vi "main.vi"() -> ()   [LabVIEW 2016]
uses:
  <vilib>/Analysis/baseanly.llb/Mean (DBL).vi
  <vilib>/Instr/_visa.llb/VISA Configure Serial Port (Instr).vi
  <vilib>/measure/mamon.llb/Waveform Peak Detection for 1 Chan.vi
  <vilib>/measure/NI_MAPro.lvlib
  <vilib>/Analysis/NI_AALBase.lvlib
panel:
  out "Heart Rate":string
  in  "Force Redraw":bool
  out "read buffer":string
  out "error out":errorcluster
  out "Value of last sample":i32
  out "Heart Rate Plot":i32(graph)
  out "Main loop interations":i32
  in  "stop":bool
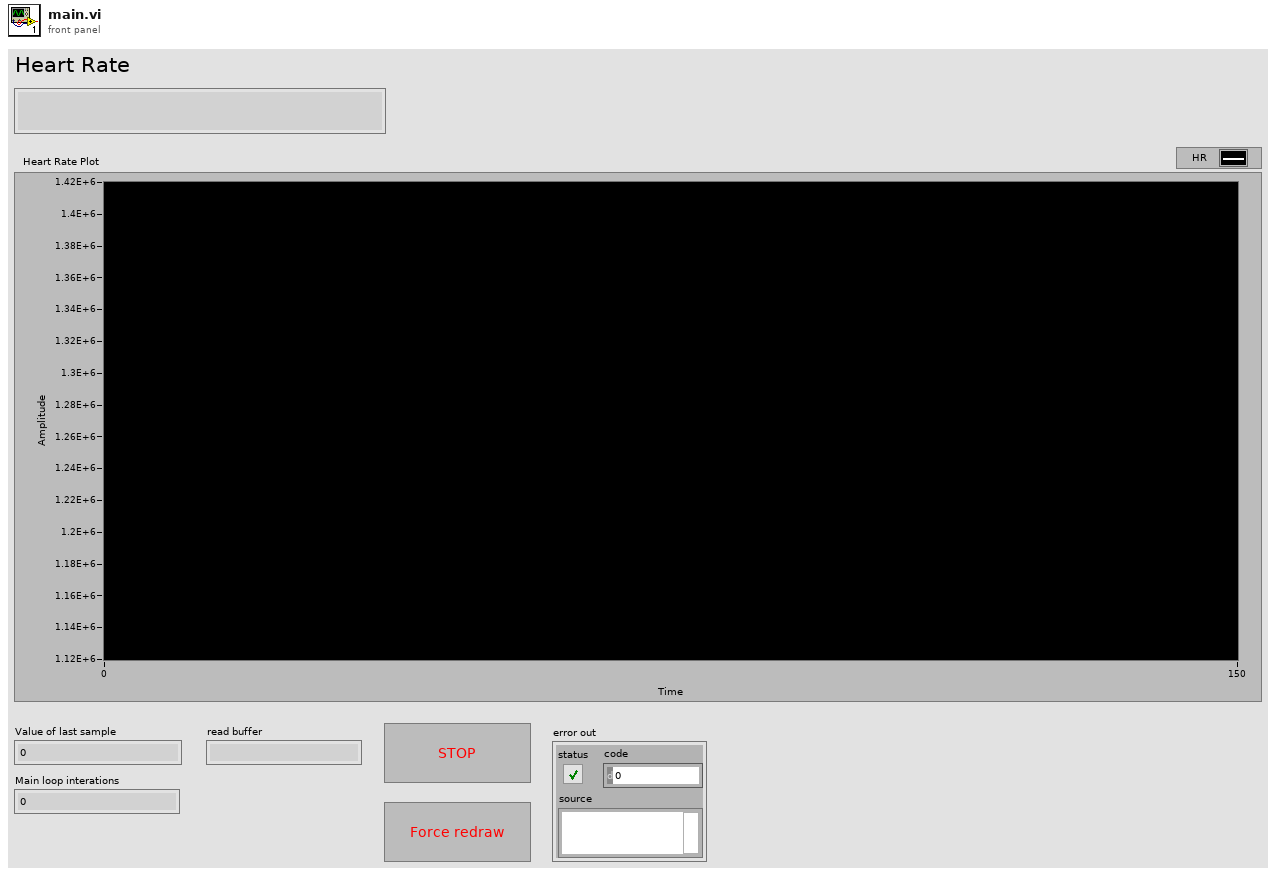
[diagram p1: front panel]
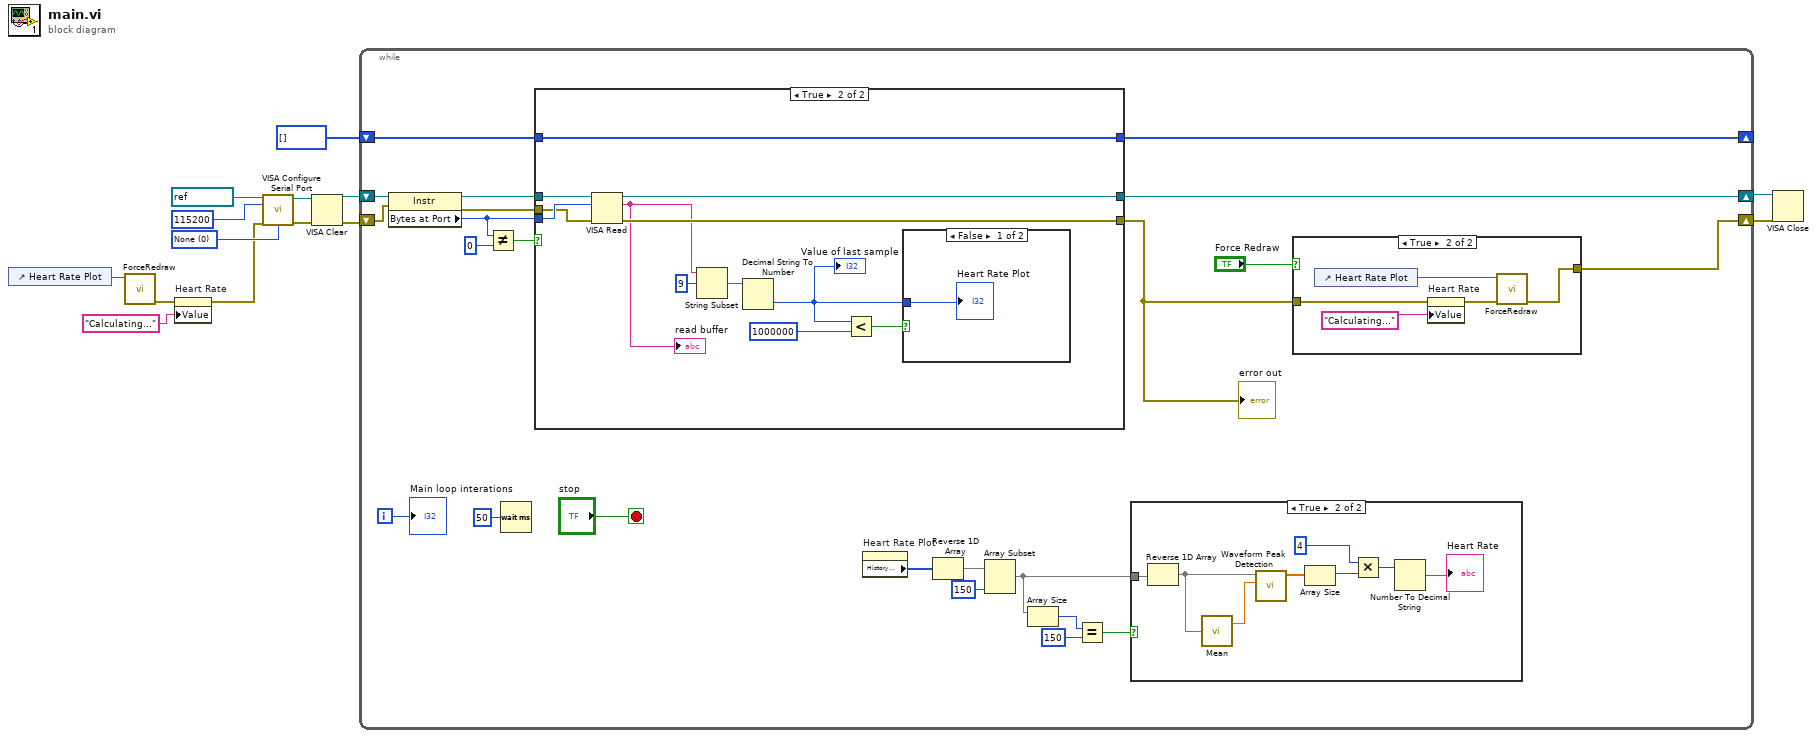
[diagram p0: block diagram]
diagram:
  w10 = u16 0 items=["None", "XON/XOFF", "RTS/CTS", "XON/XOFF & RTS/CTS", "DTR/DSR", "XON/XOFF & DTR/DSR"] ("flow control (0:none)")
  n1 = control-ref of="Heart Rate Plot"() -> (w4:refnum<vi>)
  n2 = call "ForceRedraw.vi"("Waveform Chart ref"=w4) -> ("error out"=w3:errorcluster)  [unwired: 10 in]
  n3 = property on="Heart Rate" class="Str"(error in=w3, "Value"="Calculating..." ("Heart Rate")) -> (error out=w2:errorcluster)  [unwired: 1 in, 1 out]
  n4 = call-poly "VISA Configure Serial Port"("VISA resource name"=refnum<visa-resource-name> "COM3", "baud rate (9600)"=u32 115200, "error in (no error)"=w2, "flow control (0:none)"=w10) -> ("VISA resource name out"=w7:refnum<visa-resource-name>, "error out"=w6:errorcluster)  [unwired: 10 in]
  n5 = VISA Clear(VISA resource name=w7, error in (no error)=w6) -> (VISA resource name out=w8:refnum<visa-resource-name>, error out=w9:errorcluster)
  n6 = while {
    shift-right: [w36] -> w12
    shift-left: w8 -> [w35]
    shift-right: [w23] -> w11
    shift-left: w9 -> [w33]
    shift-right: [w25] -> _
    shift-left: i32[] [] -> [w28]
    i -> [w32]
    stop <- "stop" stop-if-true
    n7 = property class="Instr"(reference=w35, error in=w33) -> (reference out=w31:refnum<visa-resource-name>, error out=w34:errorcluster, "Bytes at Port"=w27:u32)
    n8 = Not Equal?(x=w27, y=u32 0) -> (x != y?=w29:bool)
    n9 = Wait (ms)(milliseconds to wait=u32 50) -> ()  [unwired: 1 out]
    n10 = case shown="True" w29 {
      tunnel: [w54 w66] -> w36
      tunnel: w27 -> [_ w65]
      tunnel: w34 -> [w53 w64]
      tunnel: [w53 w63] -> w22
      tunnel: w31 -> [w54 w62]
      tunnel: w28 -> [w52 w55]
      tunnel: [w52 w55] -> w25
      frame False {
      }
      frame True {
        n11 = VISA Read(VISA resource name=w62, byte count=w65, error in (no error)=w64) -> (VISA resource name out=w66:refnum<visa-resource-name>, read buffer=w60:string, error out=w63:errorcluster)  [unwired: 1 out]
        "read buffer" <- w60
        n12 = String Subset(string=w60, offset (0)=9) -> (substring=w59:string)  [unwired: 1 in]
        n13 = Decimal String To Number(string=w59) -> (number=w58:i32)  [unwired: 2 in, 1 out]
        "Value of last sample" <- w58
        n14 = Less?(x=w58, y=1000000) -> (x < y?=w56:bool)
        n15 = case shown="False" w56 {
          tunnel: w58 -> [w67 _]
          frame False {
            "Heart Rate Plot" <- w67
          }
          frame True {
          }
        }
      }
    }
    "error out" <- w22
    n16 = property on="Heart Rate Plot" class="WFChart (strict)"() -> ("History Data"=w21:i32[])  [unwired: 2 in, 2 out]
    n17 = Reverse 1D Array(array=w21) -> (reversed array=w20:i32[])
    n18 = Array Subset(array=w20, length=150) -> (w17:i32[])  [unwired: 1 in]
    n19 = Array Size(array=w17) -> (size(s)=w16:i32)
    n20 = Equal?(x=w16, y=150) -> (x = y?=w18:bool)
    n21 = case shown="True" w18 {
      tunnel: w17 -> [_ w42]
      frame False {
      }
      frame True {
        n22 = Reverse 1D Array(array=w42) -> (reversed array=w41:i32[])
        n23 = call-poly <vilib>:"Mean.vi"("X"=w41) -> ("mean"=w40:dbl)  [unwired: 1 out]
        n24 = call-poly <vilib>:"Waveform Peak Detection.vi"("threshold"=w40, "Signal In"=w41) -> ("Locations"=w45:dbl[])  [unwired: 5 in, 4 out]
        n25 = Array Size(array=w45) -> (size(s)=w44:i32)
        n26 = Multiply(x=4, y=w44) -> (x*y=w39:i32)
        n27 = Number To Decimal String(number=w39) -> (decimal integer string=→"Heart Rate":string)  [unwired: 1 in]
      }
    }
    n28 = case shown="True" "Force Redraw" {
      tunnel: [w46 w50] -> w23
      tunnel: w22 -> [w46 w48]
      frame False {
      }
      frame True {
        n29 = control-ref of="Heart Rate Plot"() -> (w51:refnum<vi>)
        n30 = property on="Heart Rate" class="Str"(error in=w48, "Value"="Calculating..." ("Heart Rate")) -> (error out=w47:errorcluster)  [unwired: 1 in, 1 out]
        n31 = call "ForceRedraw.vi"("error in"=w47, "Waveform Chart ref"=w51) -> ("error out"=w50:errorcluster)  [unwired: 9 in]
      }
    }
    "Main loop interations" <- w32
  }
  n32 = VISA Close(VISA resource name=w12, error in (no error)=w11) -> ()  [unwired: 1 out]
